vi "QCP_GetDblArr.vi"(6 "Default Value":dbl, 8 "error in (no error)":errorcluster, 9 "Tuning Value":dbl[](array[numeric]), 10 "Value Name":string, 11 "QCP_DevRef_In":T1) -> (0 "error out":errorcluster, 2 "Values":dbl[](array[numeric]), 3 "QCP_DevRef_Out":T1)   [LabVIEW 2017]
uses:
  <userlib>/836-Library/System/QCP_V2/QCPSupportCode/QCP_RefNum.ctl
  <userlib>/836-Library/System/QCP_V2/QCPSupportCode/QCPData.ctl
panel:
  out "Exists?":bool
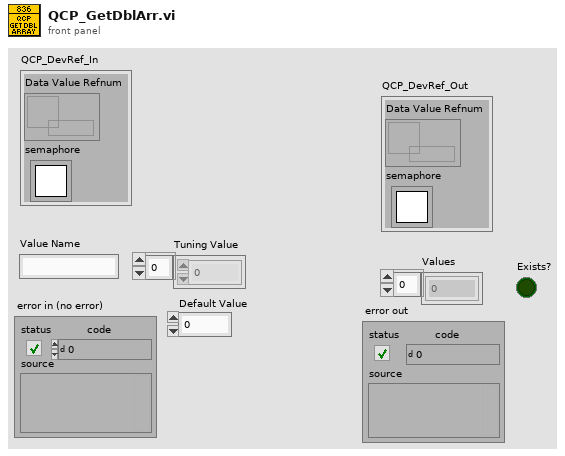
[diagram p1: front panel]
types:
  T1 = typedef "QCP_RefNum.ctl" = cluster{"Data Value Refnum":refnum<data-value>, "semaphore":T2}
  T2 = typedef "Semaphore RefNum" = refnum<k1>
  T3 = typedef "QCPData.ctl" = cluster{"Names":string[], "Values":cluster{"Array":dbl[]}[], "TuningMode?":bool}
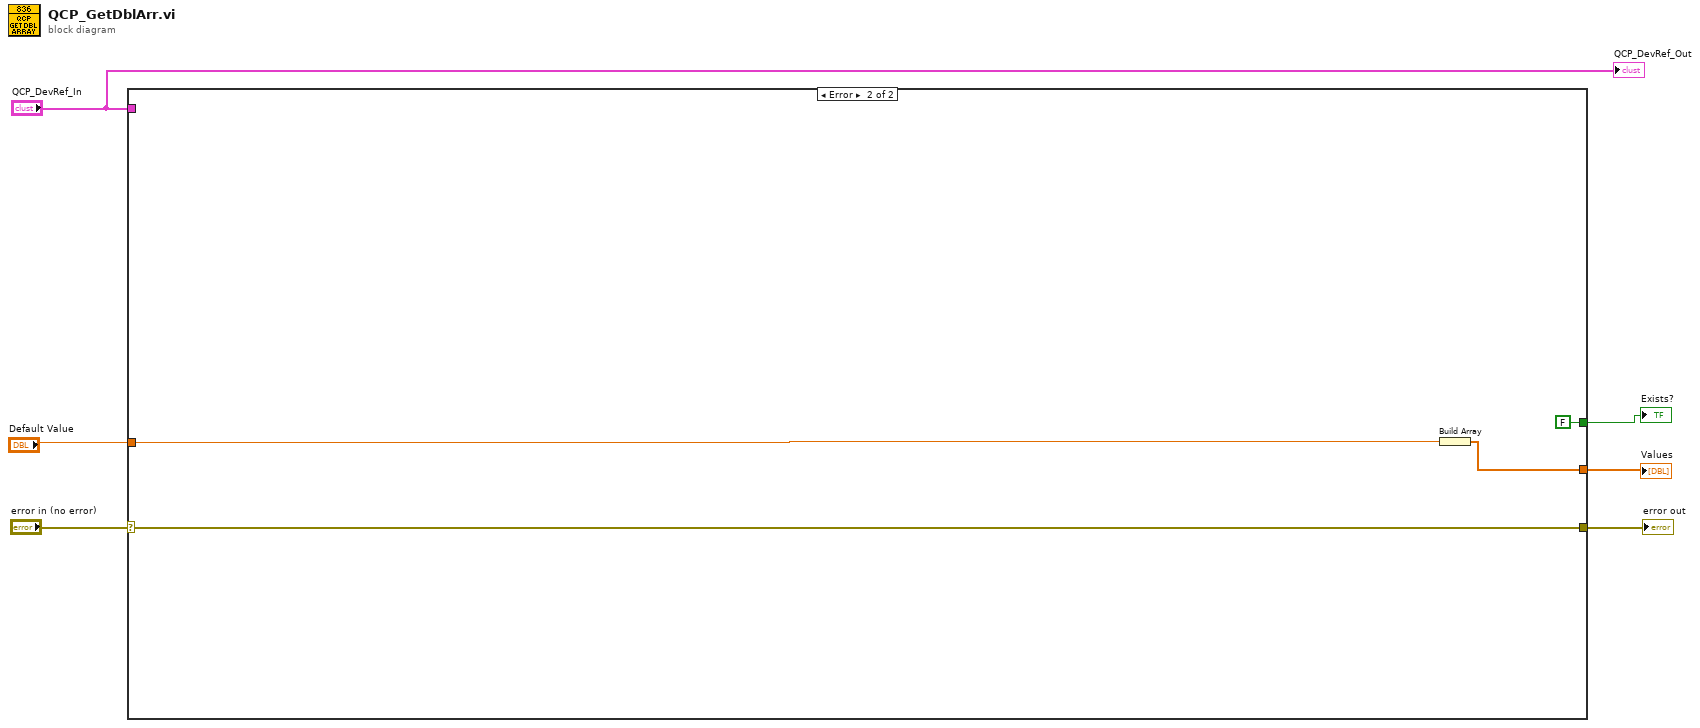
[diagram p0: block diagram]
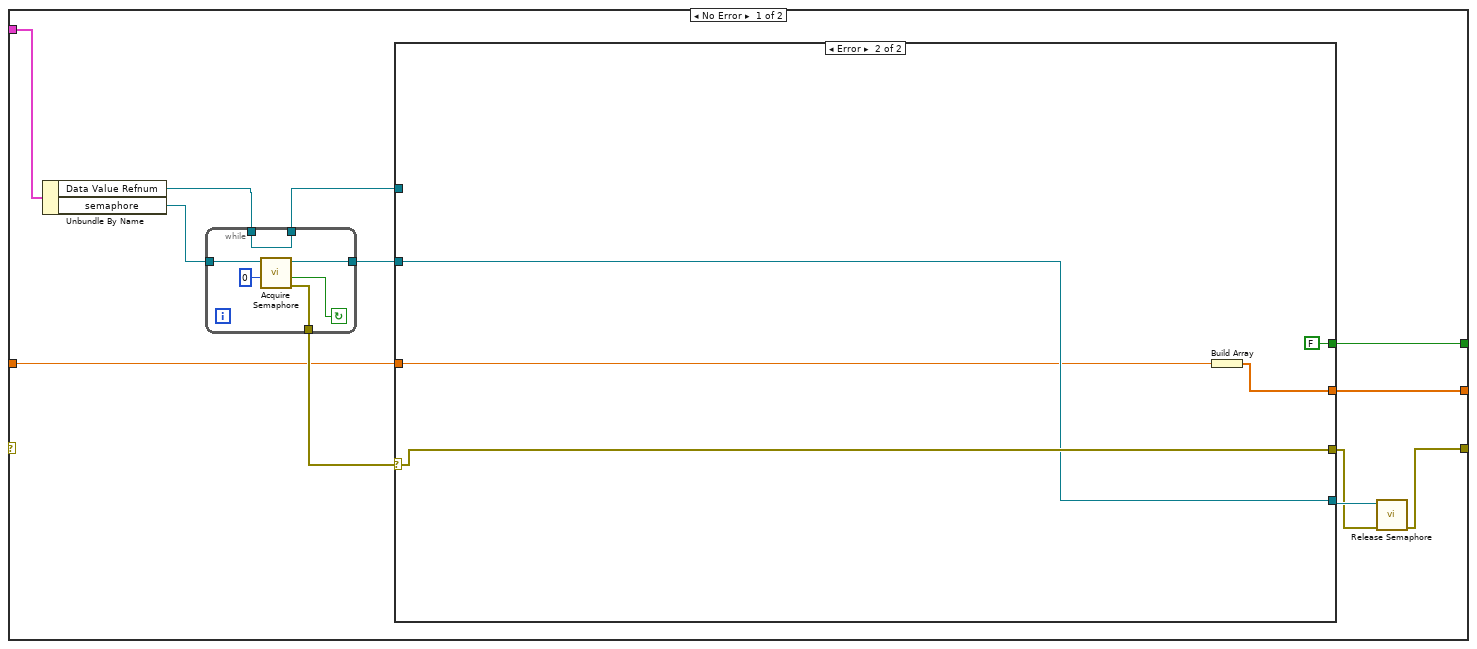
[diagram p2: hidden frame]
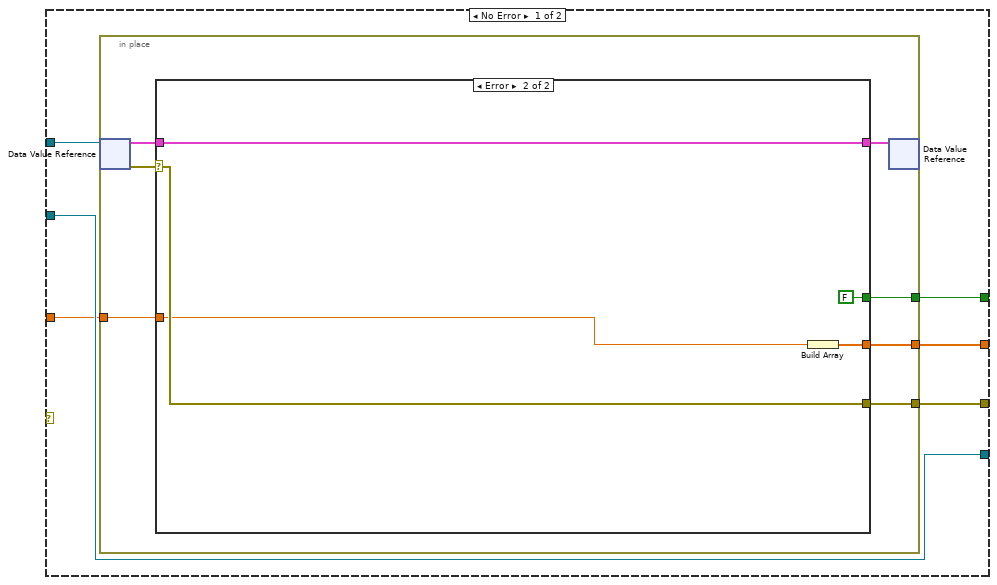
[diagram p3: hidden frame]
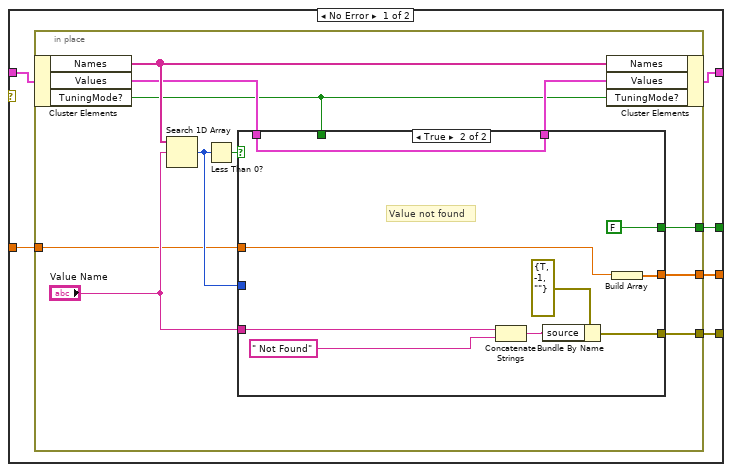
[diagram p4: hidden frame]
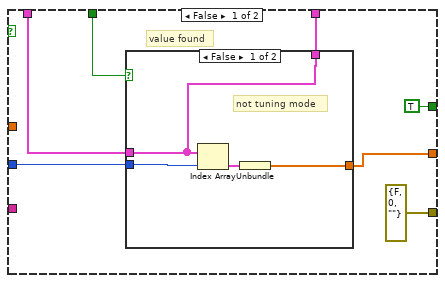
[diagram p5: hidden frame]
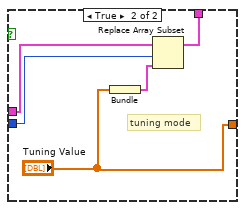
[diagram p6: hidden frame]
diagram:
  n1 = case shown="Error" "error in (no error)" {
    selector: "error in (no error)" -> [_ w93]
    tunnel: "QCP_DevRef_In" -> [w18 _]
    tunnel: [w9 w93] -> w4
    tunnel: [w17 w90] -> w3
    tunnel: [w8 FALSE] -> w2
    tunnel: "Default Value" -> [w7 w91]
    frame No Error {
      n2 = Unbundle By Name(w18) -> ("Data Value Refnum"=w15:refnum<data-value>, "semaphore"=w16:T2)
      n3 = while {
        tunnel: [w88] -> w13
        tunnel: w16 -> [w86]
        tunnel: w15 -> [w85]
        tunnel: [w85] -> w14
        tunnel: [w84] -> w12
        stop <- w89 continue-if-true
        n4 = call <vilib>:"Acquire Semaphore.vi"("ms timeout (-1)"=0, "semaphore"=w86) -> ("error out"=w88:errorcluster, "timed out"=w89:bool, "semaphore out"=w84:T2)  [unwired: 3 in]
      }
      n5 = case shown="Error" w13 {
        selector: w13 -> [_ w83]
        tunnel: [w24 w80] -> w17
        tunnel: [w23 w83] -> w10
        tunnel: w14 -> [w22 _]
        tunnel: [w21 w82] -> w11
        tunnel: w12 -> [w21 w82]
        tunnel: [w20 FALSE] -> w8
        tunnel: w7 -> [w19 w81]
        frame No Error {
          n6 = in-place {
            in-place-border: [w29] -> w24
            in-place-border: [w28] -> w23
            in-place-border: [w26] -> w20
            in-place-border: w19 -> [w25]
            n7 = in-place-dvr #1(w22) -> (w31:T3, w27:errorcluster)
            n8 = case shown="Error" w27 {
              selector: w27 -> [_ w76]
              tunnel: w31 -> [w37 w78]
              tunnel: [w36 w78] -> w30
              tunnel: [w35 w77] -> w29
              tunnel: [w34 w76] -> w28
              tunnel: [w33 FALSE] -> w26
              tunnel: w25 -> [w32 w75]
              frame No Error {
                n9 = in-place {
                  in-place-border: [w46] -> w35
                  in-place-border: [w43] -> w34
                  in-place-border: [w39] -> w33
                  in-place-border: w32 -> [w38]
                  n10 = in-place-cluster #2(w37) -> ("Names"=w48:string[], "Values"=w42:cluster{"Array":dbl[]}[], "TuningMode?"=w40:bool)
                  n11 = Search 1D Array(1D array=w48, element="Value Name") -> (index of element=w45:i32)  [unwired: 1 in]
                  n12 = Less Than 0?(x=w45) -> (x < 0?=w47:bool)
                  n13 = case shown="True" w47 {
                    tunnel: [w52 w68] -> w46
                    tunnel: w42 -> [w55 w67]
                    tunnel: w45 -> [w54 _]
                    tunnel: "Value Name" -> [_ w71]
                    tunnel: [errorcluster {"status"=FALSE, "code"=0, "source"=""} ("error constant") w69] -> w43
                    tunnel: w40 -> [w51 _]
                    tunnel: [w50 w67] -> w41
                    tunnel: [TRUE FALSE] -> w39
                    tunnel: w38 -> [_ w65]
                    frame False {
                      # "value found"
                      n14 = case shown="False" w51 {
                        tunnel: w55 -> [w56 w64]
                        tunnel: w54 -> [w58 w62]
                        tunnel: [w57 "Tuning Value"] -> w52
                        tunnel: [w56 w63] -> w50
                        frame False {
                          # "not tuning mode"
                          n15 = Index Array(array=w56, index=w58) -> (element=w59:cluster{"Array":dbl[]})
                          n16 = Unbundle(w59) -> ("Array"=w57:dbl[])
                        }
                        frame True {
                          # "tuning mode"
                          n17 = Bundle("Tuning Value"="Tuning Value") -> (w60:cluster{"Tuning Value":dbl[]})  [unwired: 1 in]
                          n18 = Replace Array Subset(array=w64, new element=w60, index=w62) -> (w63:cluster{"Array":dbl[]}[])
                        }
                      }
                    }
                    frame True {
                      # "Value not found"
                      n19 = Concatenate Strings(w71, " Not Found" ("string")) -> (w72:string)
                      n20 = Bundle By Name(cluster=errorcluster {"status"=TRUE, "code"=-1, "source"=""} ("error constant"), "source"=w72) -> (w69:errorcluster)
                      n21 = Build Array(w65) -> (w68:dbl[])
                    }
                  }
                  n22 = in-place-cluster #2("Names"=w48, "Values"=w41, "TuningMode?"=w40) -> (w36:T3)
                }
              }
              frame Error {
                n23 = Build Array(w75) -> (w77:dbl[])
              }
            }
            n24 = in-place-dvr #1(w30) -> ()  [unwired: 2 out]
          }
        }
        frame Error {
          n25 = Build Array(w81) -> (w80:dbl[])
        }
      }
      n26 = call <vilib>:"Release Semaphore.vi"("error in (no error)"=w10, "semaphore"=w11) -> ("error out"=w9:errorcluster)  [unwired: 4 in, 1 out]
    }
    frame Error {
      n27 = Build Array(w91) -> (w90:dbl[])
    }
  }
  "error out" <- w4
  "Values" <- w3
  "Exists?" <- w2
  "QCP_DevRef_Out" <- "QCP_DevRef_In"
